vi "Calculate_DS_Mean_Var.vi"(4 "PreProcessing_Options":T1={"Image Type"=4, "Normalization Type"=enum."Standardize(DS_Stats)", "Interpolation Type"=1} {"Interpolation Type" items=["Zero Order", "Bi-Linear", "Quadratic", "Cubic Spline"]; "Image Type" items=["Grayscale (U8)", "Grayscale (I16)", "Grayscale (SGL)", "Complex (CSG)", "RGB (U32)", "HSL (U32)", "RGB (U64)", "Grayscale (U16)"]}, 6 "Target Dims":T6, 8 "error in":errorcluster, 11 "File Paths":path[](array[path])) -> (0 "error out":errorcluster, 3 "Dataset_Stats":T4={"means"={"R"=0.66, "G"=0.59, "B"=0.44}, "vars"={"R"=0.66, "G"=0.59, "B"=0.44}, "DS_Size"=0} {"vars"."R" format="%#_3g"; "vars"."G" format="%#_3g"; "vars"."B" format="%#_3g"; "means"."R" format="%#_3g"; "means"."G" format="%#_3g"; "means"."B" format="%#_3g"})   [LabVIEW 2020]
uses:
  <vilib>/Ngene/Deep Learning Toolkit/Toolkit/NN_Data/API/NN_Dims(C,H,W).ctl
  PatchCore_AddOn/API/Controls/NNPC_DS_Stats.ctl
  PatchCore_AddOn/API/Controls/Image_Stats_RGB.ctl
  Controls/ImRead_PreProcessing_Options.ctl
  PatchCore_AddOn/Low_Level/Controls/Normalization_Type.ctl
  <vilib>/Analysis/NI_AALBase.lvlib
  <vilib>/vision/NI_Vision_Development_Module.lvlib
  PatchCore_AddOn/PatchCore_AddOn.lvlib
  <vilib>/Ngene/Deep Learning Toolkit/Toolkit/Deep_Learning_Toolkit_by_Ngene.lvlib
panel:
  out "iteration":i32
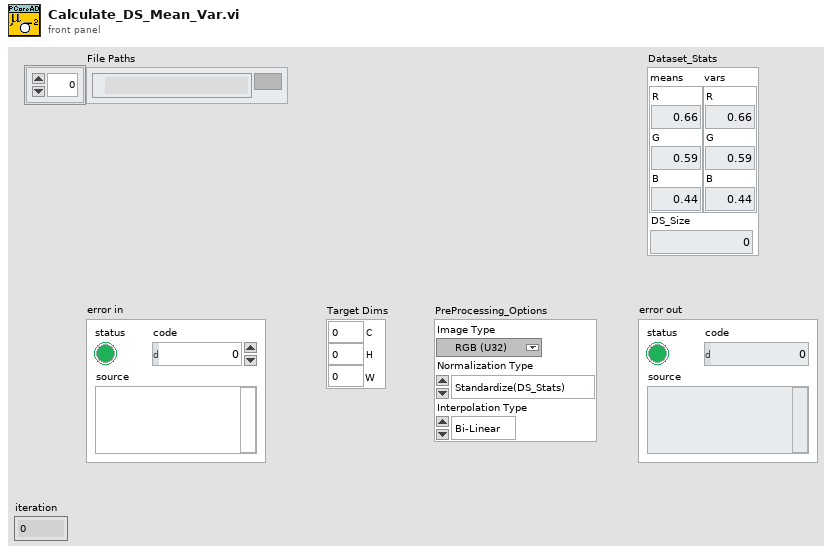
[diagram p1: front panel]
types:
  T1 = typedef "ImRead_PreProcessing_Options.ctl" = cluster{"Image Type":T2, "Normalization Type":T3, "Interpolation Type":u32}
  T2 = typedef "Image Type" = u32
  T3 = typedef "PatchCore_AddOn.lvlib/Normalization_Type.ctl" = enum16{"Standardize(DS_Stats)", "Standardize(Image_Stats)"}
  T4 = typedef "PatchCore_AddOn.lvlib/NNPC_DS_Stats.ctl" = cluster{"means":T5, "vars":T5, "DS_Size":i32}
  T5 = typedef "PatchCore_AddOn.lvlib/Image_Stats_RGB.ctl" = cluster{"R":sgl, "G":sgl, "B":sgl}
  T6 = typedef "Deep_Learning_Toolkit_by_Ngene.lvlib/NN_Dims(C,H,W).ctl" = cluster{"C":i32, "H":i32, "W":i32}
  T7 = typedef "IMAQ Image.ctl" = refnum<image>
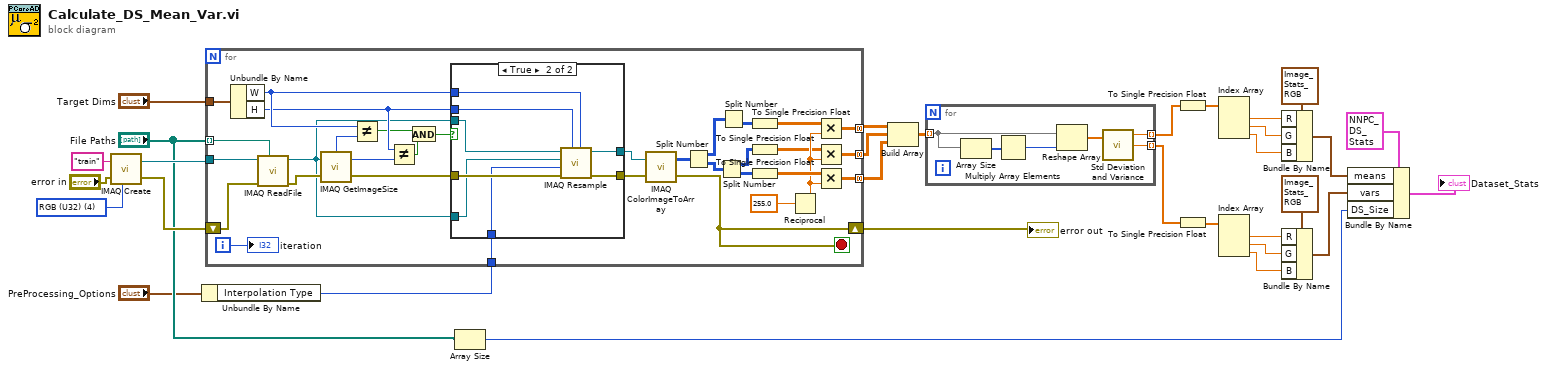
[diagram p0: block diagram]
diagram:
  w29 = T2 4 items=["Grayscale (U8)", "Grayscale (I16)", "Grayscale (SGL)", "Complex (CSG)", "RGB (U32)", "HSL (U32)", "RGB (U64)", "Grayscale (U16)"] ("Image Type")
  n1 = call "IMAQ Create"("Image Name"="train", "Image Type"=w29, "error in (no error)"="error in") -> ("New Image"=w30:T7, "error out"=w28:errorcluster)  [unwired: 2 in]
  n2 = Unbundle By Name("PreProcessing_Options") -> ("Interpolation Type"=w1:u32)
  n3 = for {
    tunnel: w30 -> [w46]
    tunnel: "File Paths" -> [w47] mode=indexing
    shift-right: [w42] -> w25
    shift-left: w28 -> [w43]
    tunnel: "Target Dims" -> [w45]
    tunnel: [w37] -> w23 mode=concatenating
    tunnel: [w36] -> w22 mode=concatenating
    tunnel: [w35] -> w21 mode=concatenating
    tunnel: w1 -> [w32]
    i -> [w41]
    stop <- w42 stop-if-true
    n4 = Unbundle By Name(w45) -> ("W"=w64:i32, "H"=w63:i32)
    n5 = call "IMAQ ReadFile"("File Path"=w47, "error in (no error)"=w43, "Image"=w46) -> ("error out"=w48:errorcluster, "Image Out"=w44:T7)  [unwired: 4 in, 3 out]
    n6 = call "IMAQ GetImageSize"("Image"=w44, "error in (no error)"=w48) -> ("Y Resolution"=w50:i32, "X Resolution"=w49:i32, "error out"=w54:errorcluster)  [unwired: 2 in]
    n7 = Not Equal?(x=w64, y=w49) -> (x != y?=w52:bool)
    n8 = Not Equal?(x=w63, y=w50) -> (x != y?=w51:bool)
    n9 = And(x=w52, y=w51) -> (x .and. y?=w53:bool)
    n10 = case shown="True" w53 {
      tunnel: w64 -> [_ w74]
      tunnel: w63 -> [_ w73]
      tunnel: [w65 w71] -> w55
      tunnel: [w66 w72] -> w56
      tunnel: w54 -> [w66 w70]
      tunnel: w44 -> [w65 w69]
      tunnel: w44 -> [_ w68]
      tunnel: w32 -> [_ w67]
      frame False {
      }
      frame True {
        n11 = call "IMAQ Resample"("X Resolution"=w74, "Y Resolution"=w73, "error in (no error)"=w70, "Interpolation Type"=w67, "Image Dst"=w68, "Image Src"=w69) -> ("error out"=w72:errorcluster, "Image Dst Out"=w71:T7)  [unwired: 4 in]
      }
    }
    n12 = call "IMAQ ColorImageToArray"("Image"=w55, "error in (no error)"=w56) -> ("Image Pixels (U32)"=w57:u32[][], "error out"=w42:errorcluster)  [unwired: 2 in, 1 out]
    n13 = Split Number(x=w57) -> (hi(x)=w59:u16[][], lo(x)=w58:u16[][])
    n14 = Split Number(x=w58) -> (hi(x)=w61:u8[][], lo(x)=w62:u8[][])
    n15 = Split Number(x=w59) -> (lo(x)=w60:u8[][])  [unwired: 1 out]
    n16 = To Single Precision Float(number=w60) -> (single precision float=w39:sgl[][])
    n17 = To Single Precision Float(number=w61) -> (single precision float=w33:sgl[][])
    n18 = To Single Precision Float(number=w62) -> (single precision float=w40:sgl[][])
    n19 = Reciprocal(x=sgl 255.0 ("y")) -> (1/x=w34:sgl)
    n20 = Multiply(x=w39, y=w34) -> (x*y=w37:sgl[][])
    n21 = Multiply(x=w33, y=w34) -> (x*y=w36:sgl[][])
    n22 = Multiply(x=w40, y=w34) -> (x*y=w35:sgl[][])
    "iteration" <- w41
  }
  "error out" <- w25
  n23 = Array Size(array="File Paths") -> (size(s)=w3:i32)
  n24 = Build Array(w23, w22, w21) -> (w20:sgl[][][])
  n25 = for {
    tunnel: [w78] -> w26 mode=indexing
    tunnel: [w77] -> w17 mode=indexing
    tunnel: w20 -> [w75] mode=indexing
    n26 = Array Size(array=w75) -> (size(s)=w80:i32[])
    n27 = Multiply Array Elements(1:w80) -> (0:w76:i32)
    n28 = Reshape Array(w75, w76) -> (w79:sgl[])
    n29 = call <vilib>:"Std Deviation and Variance.vi"("X"=w79) -> ("mean"=w78:dbl, "standard deviation"=w77:dbl)  [unwired: 1 in, 1 out]
  }
  n30 = To Single Precision Float(number=w26) -> (single precision float=w12:sgl[])
  n31 = To Single Precision Float(number=w17) -> (single precision float=w13:sgl[])
  n32 = Index Array(array=w12) -> (element #1=w11:sgl, element #2=w10:sgl, element #3=w9:sgl)  [unwired: 3 in]
  n33 = Index Array(array=w13) -> (element #1=w16:sgl, element #2=w15:sgl, element #3=w14:sgl)  [unwired: 3 in]
  n34 = Bundle By Name(cluster=T5 {"R"=0.66, "G"=0.59, "B"=0.44} ("means"), "R"=w11, "G"=w10, "B"=w9) -> (w7:T5)
  n35 = Bundle By Name(cluster=T5 {"R"=0.17, "G"=0.15, "B"=0.11} ("vars"), "R"=w16, "G"=w15, "B"=w14) -> (w5:T5)
  n36 = Bundle By Name(cluster=T4 {"means"={"R"=0.66, "G"=0.59, "B"=0.44}, "vars"={"R"=0.66, "G"=0.59, "B"=0.44}, "DS_Size"=0} ("Dataset_Stats"), "means"=w7, "vars"=w5, "DS_Size"=w3) -> (→"Dataset_Stats":T4)
